vi "src_num_lecture.vi"(11 "src":string="008") -> (1 "dN(tc)":u32[](array[numeric]), 2 "tc":dbl[](array[numeric]), 3 "tdeb":dbl[](array[numeric]), 5 "src.n":T1, 7 "src.Lib":string)   [LabVIEW 2010]
uses:
  lv_04/commandes/c0-var-n.ctl
  lv_04/lv_04.lvlib
  lv_02/lv_02.lvlib
panel:
  out "err out":errorcluster
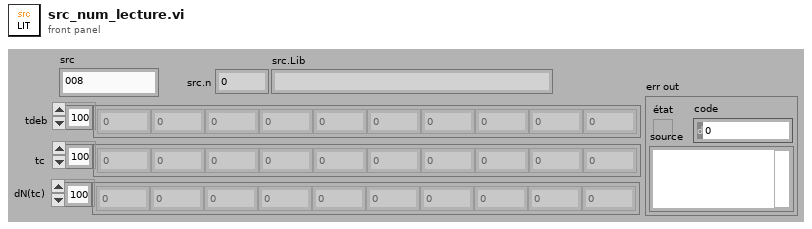
[diagram p1: front panel]
types:
  T1 = typedef "lv_04.lvlib/c0-var-n.ctl" = i32
  T2 = typedef "lv_04.lvlib/cX.ctl" = cluster{"src":T3, "num":T6, "txt":T9, "dist":T12, "Etude":enum16{"Expérimentale", "Modèle"}}
  T3 = typedef "lv_04.lvlib/cSTA_varid.ctl" = cluster{"src":string, "Lib":string, "srO":string, "V.":T4, "Voies":string[], "Do":T5, "n":T1, "Num ?":bool, "Pop ?":bool, "x_d":string, "x-u":string, "n-u":string, "MIF ?":bool}
  T4 = typedef "lv_04.lvlib/c_TDMS_ch_variable.ctl" = string
  T5 = typedef "lv_04.lvlib/c_TDMS_ch_donnees.ctl" = string
  T6 = typedef "lv_04.lvlib/cSTA_num_do_cr.ctl" = cluster{"do":T7, "sta":T8}
  T7 = typedef "lv_04.lvlib/c02-do-num.ctl" = cluster{"MIF ?":bool, "Cont. ?":bool, "xi":dbl[], "xic":dbl[], "ni":u32[], "dx":dbl[]}
  T8 = typedef "lv_04.lvlib/c04-stat-num.ctl" = cluster{"E(X)":dbl, "s":dbl, "V(X) ":dbl, "Etendue":dbl, "Mode":dbl, "Médiane":dbl}
  T9 = typedef "lv_04.lvlib/cSTA_txt_do_cr.ctl" = cluster{"do":T10, "sta":T11}
  T10 = typedef "lv_04.lvlib/c02-do-txt.ctl" = cluster{"xt":string[], "ni":dbl[], "MIF ?":bool}
  T11 = typedef "lv_04.lvlib/c04-stat-txt.ctl" = cluster{"E(X)":dbl, "s":dbl, "V(X) ":dbl, "Mode":string}
  T12 = typedef "lv_04.lvlib/cSTA_dist.ctl" = cluster{"S":T13, "T":T15, "spc":T16}
  T13 = typedef "lv_04.lvlib/c03-dist-S.ctl" = cluster{"nic":T14, "f":T14, "Fr":T14, "ni":T14}
  T14 = typedef "lv_04.lvlib/c0-dist-xy.ctl" = cluster{"x":dbl[], "y":dbl[]}
  T15 = typedef "lv_04.lvlib/c03-dist-T.ctl" = cluster{"N":T14, "Rm":T14, "R":T14, "La":T14}
  T16 = typedef "lv_04.lvlib/c03-dist-SPC.ctl" = cluster{"ech-2D":dbl[][], "ech-1D-m":dbl[], "ech-1D-s":dbl[]}
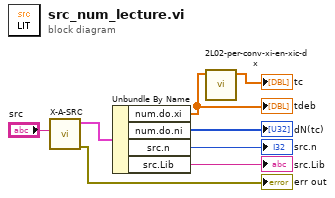
[diagram p0: block diagram]
diagram:
  n1 = call "X-A-SRC.vi"("src-nom"="src") -> ("err out"=→"err out":errorcluster, "SRC-X (s)"=w7:T2)  [unwired: 9 in]
  n2 = Unbundle By Name(w7) -> ("num.do.xi"=w6:dbl[], "num.do.ni"=→"dN(tc)":u32[], "src.n"=→"src.n":T1, "src.Lib"=→"src.Lib":string)
  "tdeb" <- w6
  n3 = call "2L02-per-conv-xi-en-xic-dx.vi"("xi"=w6) -> ("xic"=→"tc":dbl[])  [unwired: 7 in, 1 out]
